vi "GetTopMenuItem.vi"(8 "error in (no error)":errorcluster, 11 "MenuMap":map{string, T1}(c390)) -> (0 "error out":errorcluster, 2 "Item Tags":string[](array[string]), 3 "Item Names":string[](array[string]))   [LabVIEW 2021, in "Menu.lvlib" / "Menu.lvclass"]
uses:
  Menu.lvclass
  Menu.lvclass/Menu.ctl
  <vilib>/Utility/miscctls.llb/LVMenuShortCut.ctl
  MenuItems.ctl
  Picture2D/src/Picture/Image.lvclass
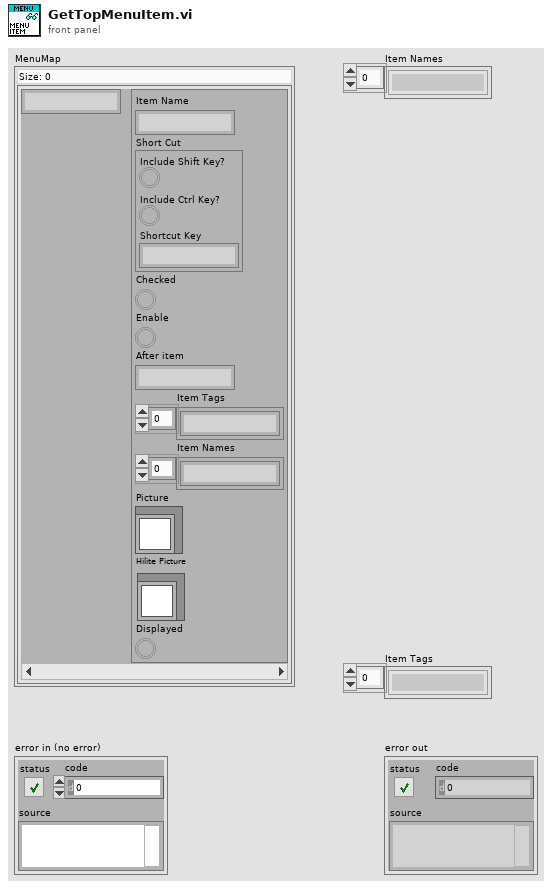
[diagram p1: front panel]
types:
  T1 = typedef "Menu.lvlib/Menu.lvclass/MenuItems.ctl" = cluster{"Item Name":string, "Short Cut":T2, "Checked":bool, "Enable":bool, "After item":string, "Item Tags":string[], "Item Names":string[], "Picture":refnum<class "Image.lvclass">, "Hilite Picture":refnum<class "Image.lvclass">, "Displayed":bool}
  T2 = typedef "LVMenuShortCut.ctl" = cluster{"Include Shift Key?":bool, "Include Ctrl Key?":bool, "Shortcut Key":string}
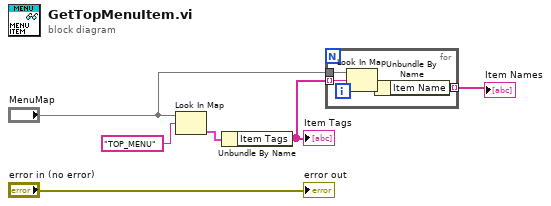
[diagram p0: block diagram]
diagram:
  n1 = Look In Map(map="MenuMap", key="TOP_MENU") -> (value=w6:T1)  [unwired: 1 in, 1 out]
  n2 = Unbundle By Name(w6) -> ("Item Tags"=w2:string[])
  "Item Tags" <- w2
  n3 = for {
    tunnel: "MenuMap" -> [w10]
    tunnel: w2 -> [w9] mode=indexing
    tunnel: [w7] -> w1 mode=indexing
    n4 = Look In Map(map=w10, key=w9) -> (value=w8:T1)  [unwired: 1 in, 1 out]
    n5 = Unbundle By Name(w8) -> ("Item Name"=w7:string)
  }
  "Item Names" <- w1
  "error out" <- "error in (no error)"
